vi "GetSensorValues.vi"(1 "Ref_BuiltInAccelerometer":T8={"DevStatus"={"status"=FALSE, "code"=0, "source"=""}, "Scaling"={"Gain (VoltsPerG)"=0.0, "Center Voltage"=0.0}, "Analog Channels"={"X-Axis"=enum."Invalid", "Y-Axis"=enum."Invalid", "Z-Axis"=enum."Invalid"}, "I2C Bus"=enum."Invalid", "SPI Bus"=enum."Invalid", "Accel Range"=0, "ADXL Axes"={"X-Axis"=FALSE, "Y-Axis"=FALSE, "Z-Axis"=FALSE}, "Handle"=0, "Device Address"=0, "Accel Type"=enum."Analog"} {"Device Address" format="%.0x"; "Accel Range" items=["+/- 2 g", "+/- 4 g", "+/- 8 g", "+/- 16 g"]}, 3 "Rear Prox Sensor":T6, 4 "Right Prox Sensor":T6, 5 "Left Prox Sensor":T6, 6 "Upper Pressure Transducer":T6, 8 "Ref_Compressor":T15, 9 "Front-Right Prox Sensor":T6, 10 "Ref_ElevatorEncoder":T1={"DeviceStatus"={"status"=FALSE, "code"=0, "source"=""}, "Type"=enum."PWM", "PWM"={"PWM Channel"=enum."Invalid", "DeadBand"={"Name"="", "maxPositivePwm"=0, "minPositivePwm"=0, "centerPwm"=0, "maxNegativePwm"=0, "minNegativePwm"=0, "angularRange"=0}}, "CAN"={"Device Number"=0, "SetOutput VI Ref"=variant, "GetOutput VI Ref"=variant, "Enable VI Ref"=variant, "Disable VI Ref"=variant, "Data"=variant}, "Invert"=FALSE, "DIO PWM"={"PWM \"Enable\" Channel"=enum."Invalid", "DIOChannel"=enum."Invalid", "PWM Rate"=0.0}}, 11 "Front-Left Prox Sensor":T6, 12 "Ref_ElevatorLimitSwitches":T1={"DeviceStatus"={"status"=FALSE, "code"=0, "source"=""}, "Type"=enum."PWM", "PWM"={"PWM Channel"=enum."Invalid", "DeadBand"={"Name"="", "maxPositivePwm"=0, "minPositivePwm"=0, "centerPwm"=0, "maxNegativePwm"=0, "minNegativePwm"=0, "angularRange"=0}}, "CAN"={"Device Number"=0, "SetOutput VI Ref"=variant, "GetOutput VI Ref"=variant, "Enable VI Ref"=variant, "Disable VI Ref"=variant, "Data"=variant}, "Invert"=FALSE, "DIO PWM"={"PWM \"Enable\" Channel"=enum."Invalid", "DIOChannel"=enum."Invalid", "PWM Rate"=0.0}}, 15 "Tank Pressure Transducer":T6, 19 "Ground Prox Sensor":T6, 20 "Ref_Drive 1R":T1, 21 "Ref_Drive 2R":T1, 22 "Ref_Drive 3L":T1, 23 "Ref_Drive 4L":T1, 24 "Ref_Drive 5L":T1, 26 "Ref_Drive 6R":T1) -> ()   [LabVIEW 2018]
uses:
  <vilib>/Rock Robotics/WPI/AnalogChannel/WPI_AnalogChannelDevRef.ctl
  <vilib>/Rock Robotics/SystemInterfaces/AI/FPGA_AIChannel.ctl
  <vilib>/Rock Robotics/WPI/Compressor/WPI_CompressorDevRef.ctl
  <vilib>/Rock Robotics/WPI/MotorControl/WPI_MotorControlDeviceRef.ctl
  <vilib>/Rock Robotics/WPI/MotorControl/WPI_MotorControlType.ctl
  <vilib>/Rock Robotics/SystemInterfaces/DIO/FPGA_DIOPWMChannel.ctl
  <vilib>/Rock Robotics/WPI/PWM/WPI_PWMDeadband.ctl
  <vilib>/Rock Robotics/SystemInterfaces/DIO/FPGA_DIOChannel.ctl
  <vilib>/Rock Robotics/WPI/Accelerometer/WPI_AccelerometerDevRef.ctl
  <vilib>/Rock Robotics/WPI/Accelerometer/WPI_AccelerometerScaling.ctl
  <vilib>/Rock Robotics/WPI/Accelerometer/WPI_AccelerometerAnalogChannels.ctl
  <vilib>/Rock Robotics/SystemInterfaces/i2clib/i2c_bus.ctl
  <vilib>/Rock Robotics/SystemInterfaces/spilib/spi_bus.ctl
  <vilib>/Rock Robotics/WPI/Accelerometer/ADXL345 Range.ctl
  <vilib>/Rock Robotics/WPI/Accelerometer/WPI_AccelerometerADXL345 Axes.ctl
  SensorReadings.vi
  RefNums_Actuators.vi
  RobotStates.vi
  Inputs_DriverStation.vi
  <vilib>/Rock Robotics/WPI/ThirdParty/Phoenix-LabVIEW/Motor Controller/Get/CTRE_Phoenix_MotorController_GetLimitSwitchStates.vi
  <vilib>/Rock Robotics/WPI/ThirdParty/Phoenix-LabVIEW/Motor Controller/Get/CTRE_Phoenix_MotorController_GetSelectedSensorData.vi
  <vilib>/gmath/NI_Gmath.lvlib
  <vilib>/Analysis/NI_AALBase.lvlib
panel:
  in  "Normal Elevator Std (A)":dbl=35.0
  in  "Off Ground Time (ms)":u32=100
  in  "On Ground Time (ms)":u32=1000
  in  "Ground Distance (in)":dbl=6.0
  in  "Plot Drive Encoder Data":bool
  in  "Tank Pressure Voltage Table":dbl[](array[numeric])=[0.4, 0.7, 0.9, 1.2, 1.4, 1.7, 1.9, 2.3, 2.5, 2.8, 3.0, 3.3] format="%_6g"
  in  "Tank Pressure PSI Table":dbl[](array[numeric])=[0.0, 10.0, 20.0, 30.0, 40.0, 50.0, 60.0, 70.0, 80.0, 90.0, 100.0, 115.0] format="%_6g"
  in  "LR Voltage Table":dbl[](array[numeric])=[0.43, 0.45, 0.47, 0.55, 0.6, 0.68, 0.72, 0.81, 0.86, 0.98, 1.13, 1.36, 1.53, 1.77, 1.99, 2.26, 2.52, 2.76] format="%_6g"
  in  "LR Distance Table":dbl[](array[numeric])=[150.661, 140.6, 133.7, 120.9, 110.1, 95.3, 90.1, 80.0, 73.7, 64.6, 55.9, 45.6, 40.2, 35.0, 29.6, 24.3, 19.6, 14.8] format="%_6g"
  in  "Suction Threshold (V)":dbl=0.1
  in  "SR Voltage Table":dbl[](array[numeric])=[3.15, 2.82, 2.51, 2.16, 1.92, 1.7, 1.49, 1.3, 1.12, 0.97, 0.87, 0.79, 0.72, 0.64, 0.61, 0.58, 0.52, 0.47, 0.46, 0.45, 0.43, 0.41] format="%_6g"
  in  "SR Distance Table":dbl[](array[numeric])=[4.6, 6.6, 8.3, 10.4, 12.2, 14.1, 16.5, 19.9, 23.6, 28.2, 32.6, 36.8, 40.9, 46.3, 49.9, 53.7, 58.3, 63.5, 67.5, 71.5, 75.1, 78.9] format="%_6g"
  out "Drive Encoder Velocities":cluster{dbl, dbl}(graph)
  # "*** Alpha was set to 6 inches ***"
  # "*** Beta was set to 12 inches ***"
  # "ADXL"
  # "Analog"
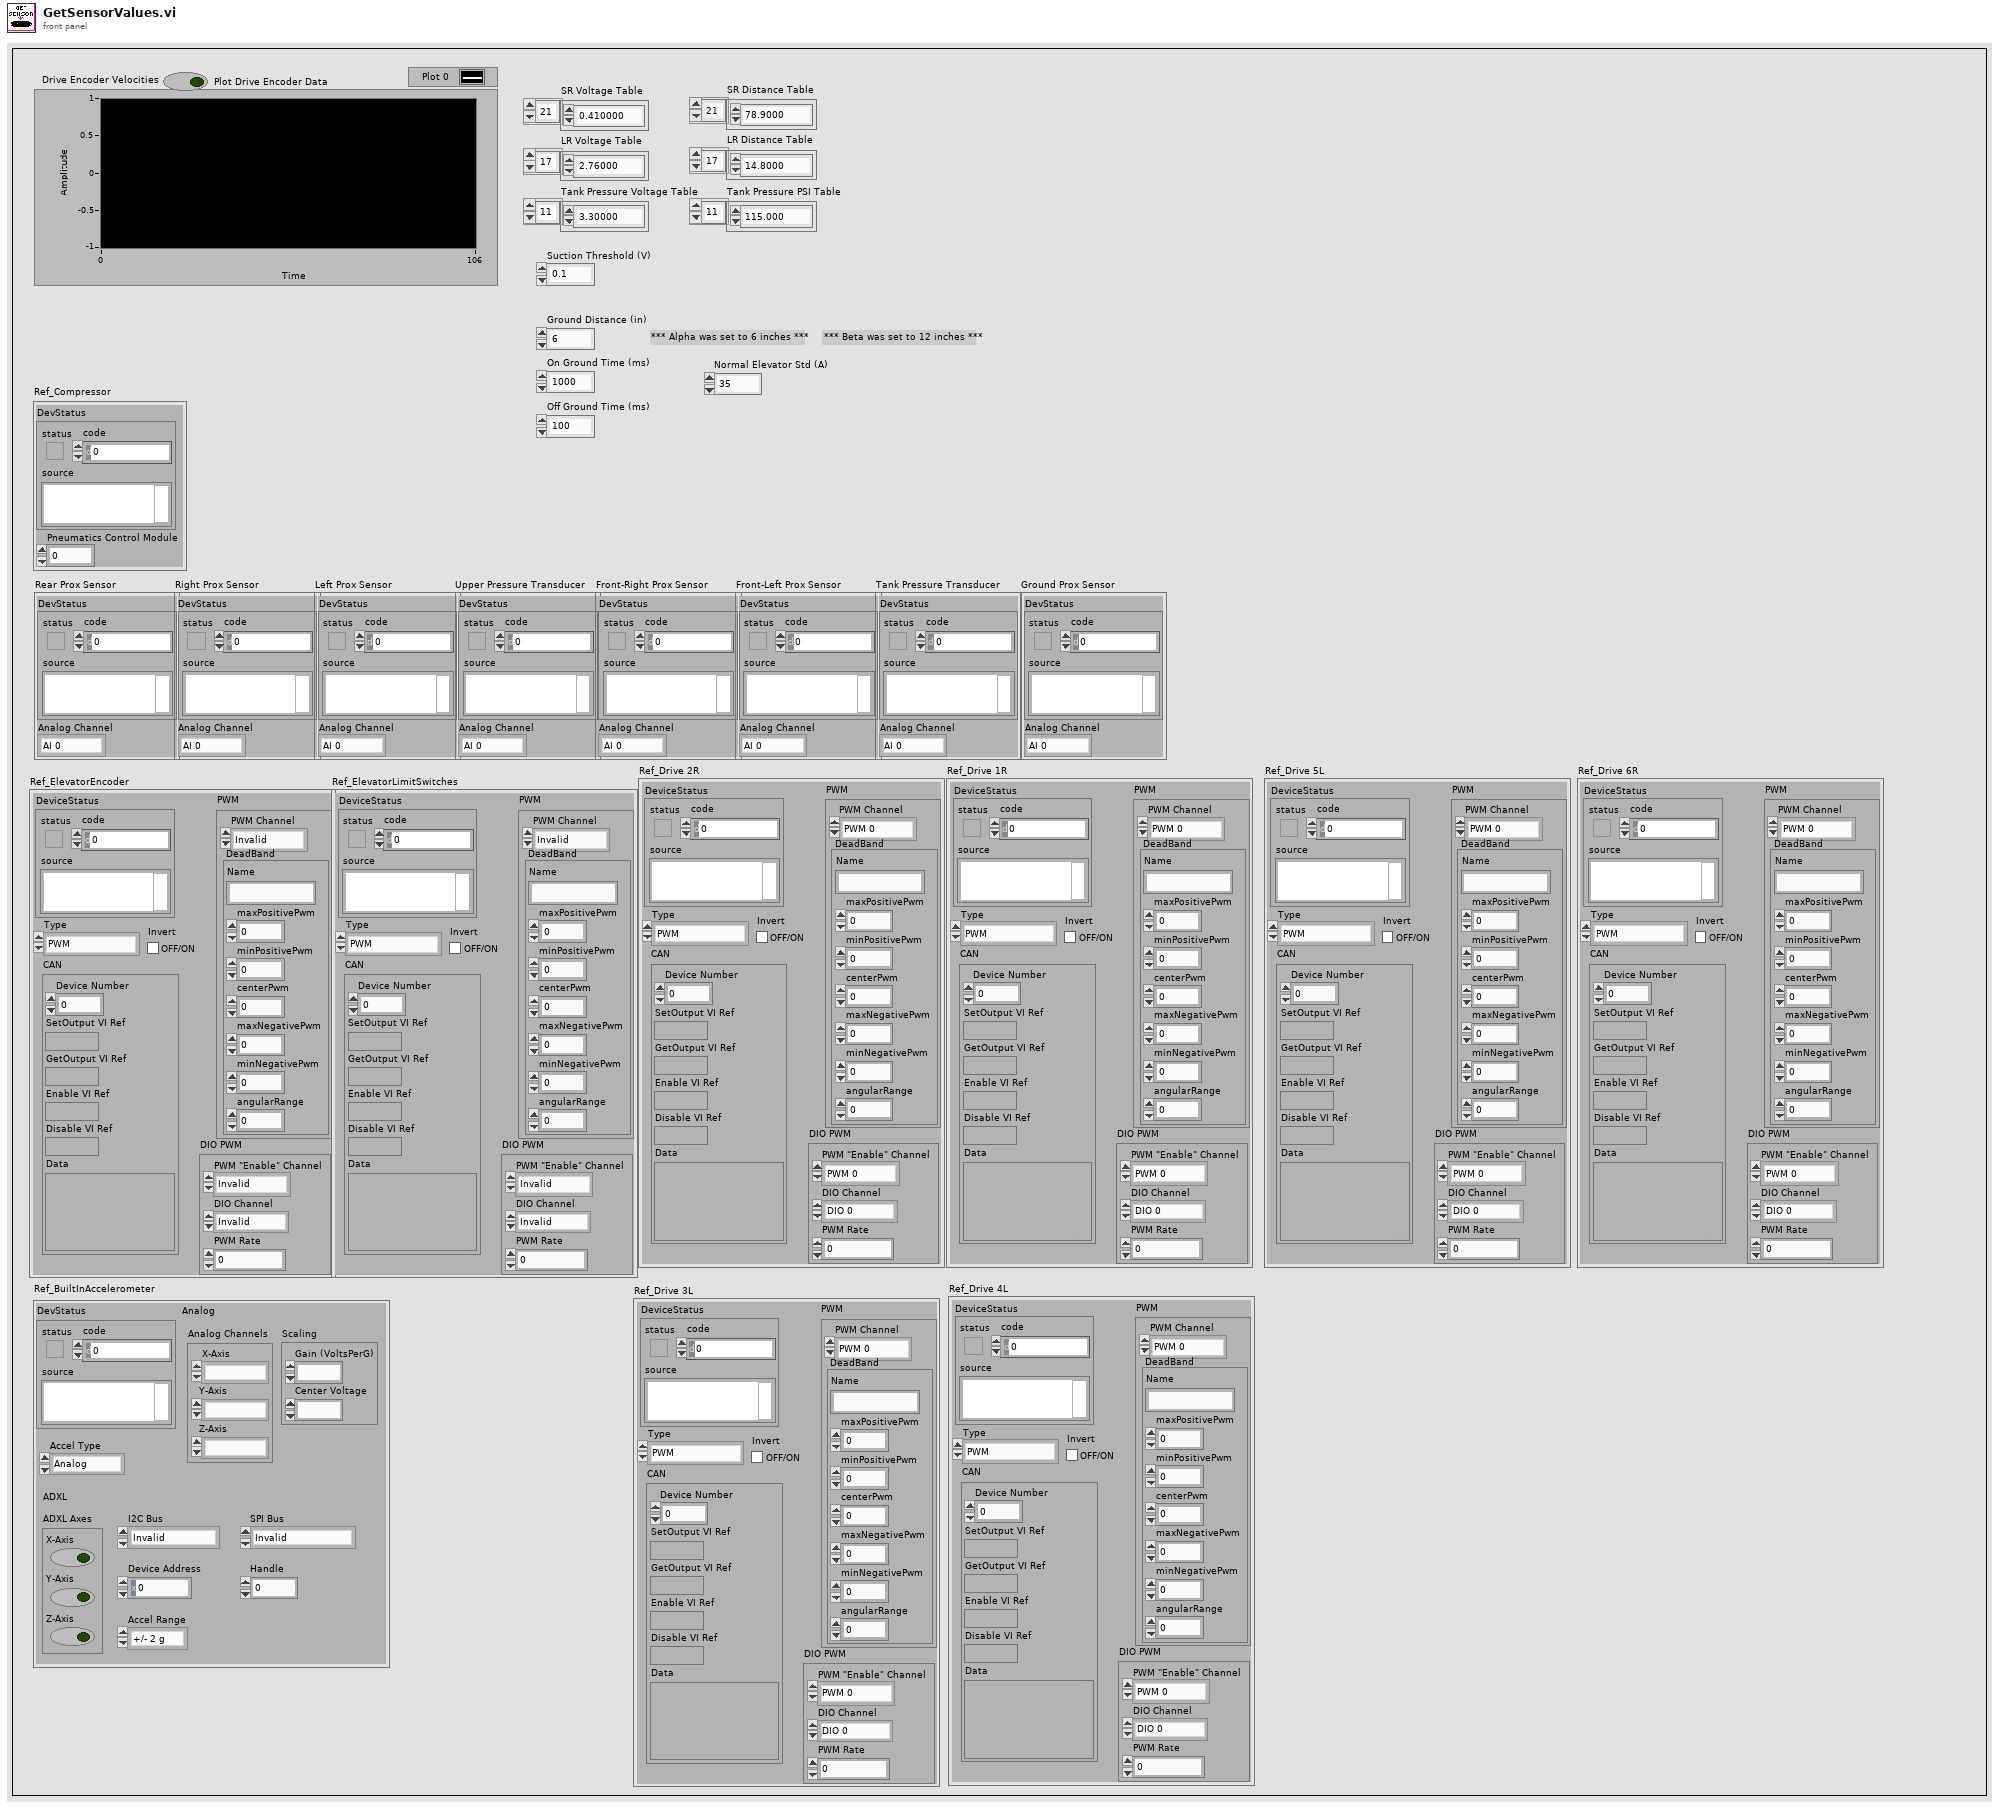
[diagram p1: front panel]
types:
  T1 = typedef "WPI_MotorControlDeviceRef.ctl" = cluster{"DeviceStatus":errorcluster, "Type":T2, "PWM":cluster{"PWM Channel":T3, "DeadBand":T4}, "CAN":cluster{"Device Number":u8, "SetOutput VI Ref":variant, "GetOutput VI Ref":variant, "Enable VI Ref":variant, "Disable VI Ref":variant, "Data":variant}, "Invert":bool, "DIO PWM":cluster{"PWM \"Enable\" Channel":T3, "DIOChannel":T5, "PWM Rate":dbl}}
  T2 = typedef "WPI_MotorControlType.ctl" = enum16{"PWM", "CAN", "DIO PWM"}
  T3 = typedef "FPGA_DIOPWMChannel.ctl" = enum8{"PWM 0", "PWM 1", "PWM 2", "PWM 3", "PWM 4", "PWM 5", "PWM 6", "PWM 7", "PWM 8", "PWM 9", "PWM MXP 0", "PWM MXP 1", "PWM MXP 2", "PWM MXP 3", "PWM MXP 4", "PWM MXP 5", "PWM MXP 6", "PWM MXP 7", "PWM MXP 8", "PWM MXP 9", "Invalid"}
  T4 = typedef "WPI_PWMDeadband.ctl" = cluster{"Name":string, "maxPositivePwm":i32, "minPositivePwm":i32, "centerPwm":i32, "maxNegativePwm":i32, "minNegativePwm":i32, "angularRange":u16}
  T5 = typedef "FPGA_DIOChannel.ctl" = enum8{"DIO 0", "DIO 1", "DIO 2", "DIO 3", "DIO 4", "DIO 5", "DIO 6", "DIO 7", "DIO 8", "DIO 9", "DIO MXP 0", "DIO MXP 1", "DIO MXP 2", "DIO MXP 3", "DIO MXP 4", "DIO MXP 5", "DIO MXP 6", "DIO MXP 7", "DIO MXP 8", "DIO MXP 9", "DIO MXP 10", "DIO MXP 11", "DIO MXP 12", "DIO MXP 13", "DIO MXP 14", "DIO MXP 15", "SPI Port CS1", "SPI Port CS2", "SPI Port CS3", "SPI Port MISO", "SPI Port MOSI", "Invalid"}
  T6 = typedef "WPI_AnalogChannelDevRef.ctl" = cluster{"DevStatus":errorcluster, "Analog Channel":T7}
  T7 = typedef "FPGA_AIChannel.ctl" = enum8{"AI 0", "AI 1", "AI 2", "AI 3", "AI MXP 0", "AI MXP 1", "AI MXP 2", "AI MXP 3", "Invalid"}
  T8 = typedef "WPI_AccelerometerDevRef.ctl" = cluster{"DevStatus":errorcluster, "Scaling":T9, "Analog Channels":T10, "I2C Bus":T11, "SPI Bus":T12, "Accel Range":T13, "ADXL Axes":T14, "Handle":i32, "Device Address":u8, "Accel Type":enum16{"Analog", "ADXL345 I2C", "ADXL345 SPI", "Internal", "ADXL362 SPI"}}
  T9 = typedef "WPI_AccelerometerScaling.ctl" = cluster{"Gain (VoltsPerG)":dbl, "Center Voltage":dbl}
  T10 = typedef "WPI_AccelerometerAnalogChannels.ctl" = cluster{"X-Axis":T7, "Y-Axis":T7, "Z-Axis":T7}
  T11 = typedef "i2c_bus.ctl" = enum16{"I2C On-Board", "I2C MXP", "Invalid"}
  T12 = typedef "spi_bus.ctl" = enum16{"SPI On-Board, CS0", "SPI On-Board, CS1", "SPI On-Board, CS2", "SPI On-Board, CS3", "SPI MXP", "Invalid"}
  T13 = typedef "ADXL345 Range.ctl" = u8
  T14 = typedef "WPI_AccelerometerADXL345 Axes.ctl" = cluster{"X-Axis":bool, "Y-Axis":bool, "Z-Axis":bool}
  T15 = typedef "WPI_CompressorDevRef.ctl" = cluster{"DevStatus":errorcluster, "Pneumatics Control Module":u8}
  T16 = cluster{"X-Axis":dbl, "Y-Axis":dbl, "Z-Axis":dbl}
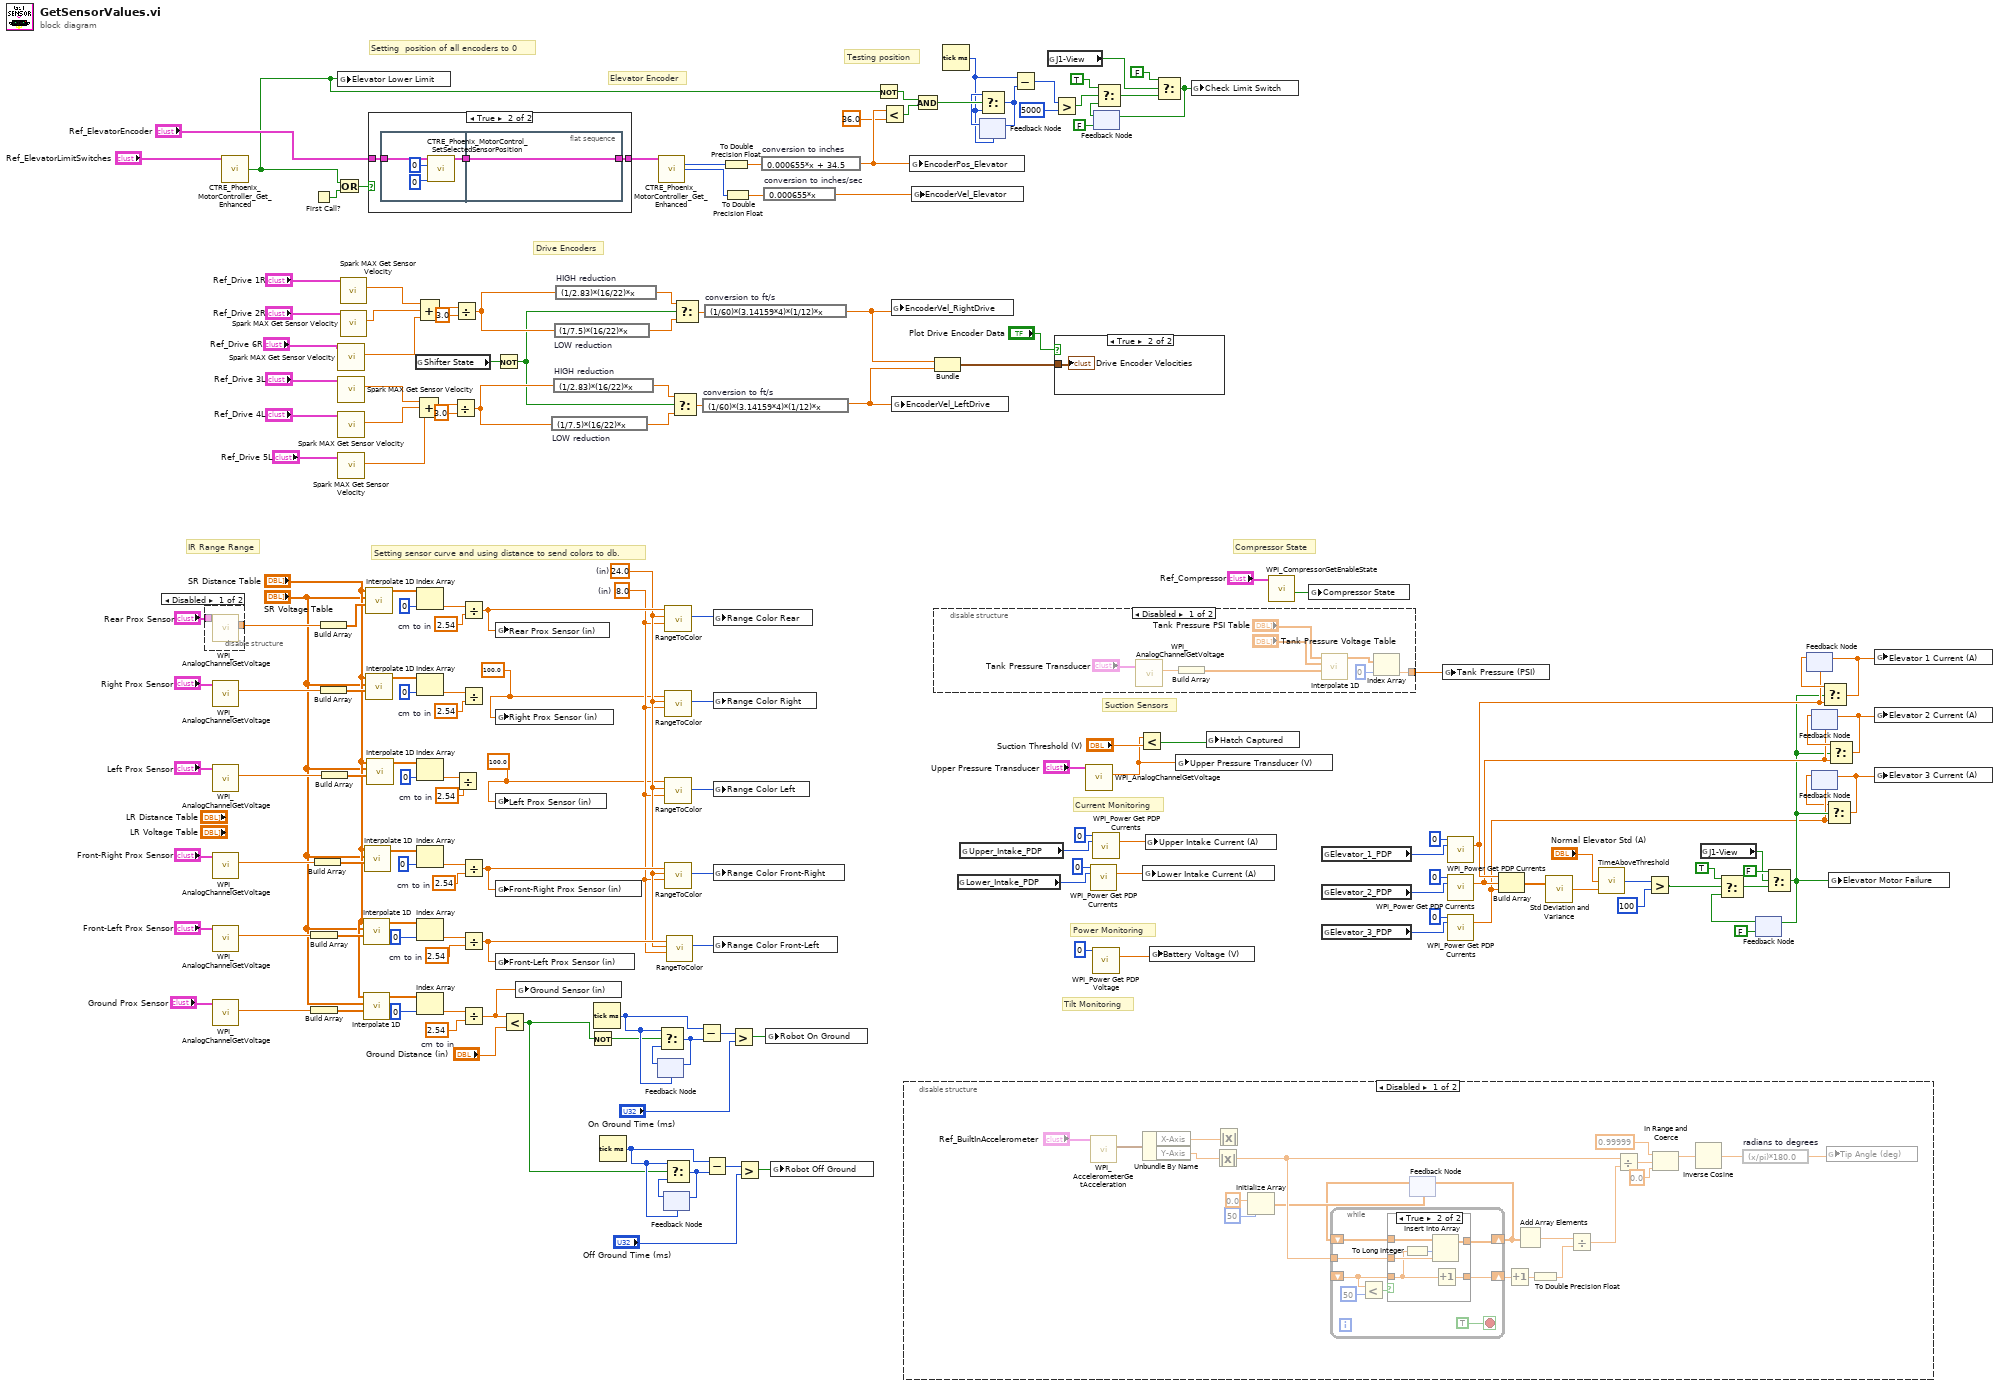
[diagram p0: block diagram]
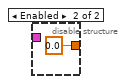
[diagram p2: hidden frame]
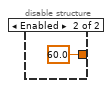
[diagram p6: hidden frame]
diagram:
  w5 = 100.0
  w6 = 100.0
  w76 = 2.54  # cm to in
  w133 = 2.54  # cm to in
  w126 = 8.0  # (in)
  w127 = 24.0  # (in)
  w150 = 2.54  # cm to in
  w156 = 2.54  # cm to in
  w163 = 2.54  # cm to in
  w170 = 2.54  # cm to in
  # "Elevator Encoder"
  # "Tilt Monitoring"
  # "Drive Encoders"
  # "Power Monitoring"
  # "Testing position"
  # "Setting  position of all encoders to 0"
  # "Setting sensor curve and using distance to send colors to db."
  # "Current Monitoring"
  # "Suction Sensors"
  # "Compressor State"
  # "IR Range Range"
  n1 = disable-structure shown="Disabled" {
    disable-tunnel: [w176 0.0 ("Voltage")] -> w174
    disable-tunnel: "Rear Prox Sensor" -> [w175 _]
    frame Disabled {
      n2 = call <vilib>:"WPI_AnalogChannelGetVoltage.vi"("AIDeviceRef"=w175) -> ("Voltage"=w176:dbl)  [unwired: 8 in, 2 out]
    }
    frame Enabled {
    }
  }
  n3 = call <vilib>:"WPI_AnalogChannelGetVoltage.vi"("AIDeviceRef"="Right Prox Sensor") -> ("Voltage"=w168:dbl)  [unwired: 8 in, 2 out]
  n4 = call <vilib>:"WPI_AnalogChannelGetVoltage.vi"("AIDeviceRef"="Left Prox Sensor") -> ("Voltage"=w161:dbl)  [unwired: 8 in, 2 out]
  n5 = call <vilib>:"WPI_AnalogChannelGetVoltage.vi"("AIDeviceRef"="Front-Right Prox Sensor") -> ("Voltage"=w138:dbl)  [unwired: 8 in, 2 out]
  n6 = call <vilib>:"WPI_AnalogChannelGetVoltage.vi"("AIDeviceRef"="Front-Left Prox Sensor") -> ("Voltage"=w131:dbl)  [unwired: 8 in, 2 out]
  n7 = call <vilib>:"WPI_AnalogChannelGetVoltage.vi"("AIDeviceRef"="Ground Prox Sensor") -> ("Voltage"=w75:dbl)  [unwired: 8 in, 2 out]
  n8 = call-poly <vilib>:"CTRE_Phoenix_MotorController_Get_Enhanced.vi"("PhoenixMotorControlDevRef"="Ref_ElevatorLimitSwitches") -> ("Reverse Limit Closed?"=w22:bool)  [unwired: 11 in, 3 out]
  n9 = First Call?() -> (First Call?: T/F=w80:bool)
  n10 = Build Array(w131) -> (w136:dbl[])
  n11 = Build Array(w75) -> (w79:dbl[])
  n12 = Build Array(w138) -> (w154:dbl[])
  n13 = Build Array(w174) -> (w148:dbl[])
  n14 = Build Array(w168) -> (w167:dbl[])
  n15 = Build Array(w161) -> (w160:dbl[])
  n16 = Or(x=w22, y=w80) -> (x .or. y?=w81:bool)
  n17 = global write "SensorReadings.vi" "Elevator Lower Limit"(w22) -> ()
  n18 = call <vilib>:"Spark MAX Get Sensor Velocity.vi"("MotorControlDevRef in"="Ref_Drive 6R") -> ("Sensor Velocity"=w2:dbl)  [unwired: 7 in, 3 out]
  n19 = call <vilib>:"Spark MAX Get Sensor Velocity.vi"("MotorControlDevRef in"="Ref_Drive 3L") -> ("Sensor Velocity"=w108:dbl)  [unwired: 7 in, 3 out]
  n20 = call <vilib>:"Spark MAX Get Sensor Velocity.vi"("MotorControlDevRef in"="Ref_Drive 4L") -> ("Sensor Velocity"=w107:dbl)  [unwired: 7 in, 3 out]
  n21 = call <vilib>:"Spark MAX Get Sensor Velocity.vi"("MotorControlDevRef in"="Ref_Drive 5L") -> ("Sensor Velocity"=w1:dbl)  [unwired: 7 in, 3 out]
  n22 = call <vilib>:"Spark MAX Get Sensor Velocity.vi"("MotorControlDevRef in"="Ref_Drive 1R") -> ("Sensor Velocity"=w113:dbl)  [unwired: 7 in, 3 out]
  n23 = call <vilib>:"Spark MAX Get Sensor Velocity.vi"("MotorControlDevRef in"="Ref_Drive 2R") -> ("Sensor Velocity"=w54:dbl)  [unwired: 7 in, 3 out]
  n24 = call <vilib>:"Interpolate 1D.vi"("xi"=w136, "X"="SR Voltage Table", "Y"="SR Distance Table") -> ("yi"=w130:dbl[])  [unwired: 6 in, 2 out]
  n25 = call <vilib>:"Interpolate 1D.vi"("xi"=w79, "X"="SR Voltage Table", "Y"="SR Distance Table") -> ("yi"=w74:dbl[])  [unwired: 6 in, 2 out]
  n26 = call <vilib>:"Interpolate 1D.vi"("xi"=w154, "X"="SR Voltage Table", "Y"="SR Distance Table") -> ("yi"=w151:dbl[])  [unwired: 6 in, 2 out]
  n27 = call <vilib>:"Interpolate 1D.vi"("xi"=w148, "X"="SR Voltage Table", "Y"="SR Distance Table") -> ("yi"=w171:dbl[])  [unwired: 6 in, 2 out]
  n28 = call <vilib>:"Interpolate 1D.vi"("xi"=w167, "X"="SR Voltage Table", "Y"="SR Distance Table") -> ("yi"=w164:dbl[])  [unwired: 6 in, 2 out]
  n29 = call <vilib>:"Interpolate 1D.vi"("xi"=w160, "X"="SR Voltage Table", "Y"="SR Distance Table") -> ("yi"=w157:dbl[])  [unwired: 6 in, 2 out]
  n30 = case shown="True" w81 {
    tunnel: "Ref_ElevatorEncoder" -> [w178 w181]
    tunnel: [w178 w179] -> w86
    frame False {
    }
    frame True {
      n31 = flat-sequence {
        tunnel: w181 -> [w185]
        tunnel: [w184] -> w180
        tunnel: [w186] -> w179
        tunnel: w180 -> [w186]
        frame #0 {
          n32 = call <vilib>:"CTRE_Phoenix_MotorControl_SetSelectedSensorPosition.vi"("pidLoopIdx"=u32 0, "New Sensor Position"=0, "PhoenixMotorControlDevRef"=w185) -> ("PhoenixMotorControlDevRef"=w184:T1)  [unwired: 7 in, 1 out]
        }
        frame #1 {
        }
      }
    }
  }
  n33 = global read "RobotStates.vi" "Shifter State"() -> (w100:bool)
  n34 = Index Array(array=w171, index=0) -> (element=w172:dbl)
  n35 = Index Array(array=w164, index=0) -> (element=w165:dbl)
  n36 = Index Array(array=w157, index=0) -> (element=w158:dbl)
  n37 = Index Array(array=w151, index=0) -> (element=w152:dbl)
  n38 = Index Array(array=w130, index=0) -> (element=w134:dbl)
  n39 = Index Array(array=w74, index=0) -> (element=w77:dbl)
  n40 = Compound Arithmetic op=ADD(w108, w107, w1) -> (w110:dbl)
  n41 = Compound Arithmetic op=ADD(w113, w54, w2) -> (w112:dbl)
  n42 = Divide(x=w110, y=3.0) -> (x/y=w101:dbl)
  n43 = Divide(x=w112, y=3.0) -> (x/y=w104:dbl)
  n44 = Divide(x=w158, y=w156) -> ()  [unwired: 1 out]
  n45 = Divide(x=w172, y=w170) -> (x/y=w147:dbl)
  n46 = Divide(x=w165, y=w163) -> ()  [unwired: 1 out]
  n47 = Divide(x=w152, y=w150) -> (x/y=w146:dbl)
  n48 = Divide(x=w134, y=w133) -> (x/y=w132:dbl)
  n49 = Divide(x=w77, y=w76) -> (x/y=w57:dbl)
  n50 = Not(x=w100) -> (.not. x?=w88:bool)
  n51 = global write "SensorReadings.vi" "Rear Prox Sensor (in)"(w147) -> ()
  n52 = global write "SensorReadings.vi" "Right Prox Sensor (in)"(w6) -> ()
  n53 = global write "SensorReadings.vi" "Left Prox Sensor (in)"(w5) -> ()
  n54 = global write "SensorReadings.vi" "Front-Right Prox Sensor (in)"(w146) -> ()
  n55 = global write "SensorReadings.vi" "Front-Left Prox Sensor (in)"(w132) -> ()
  n56 = Less?(x=w57, y="Ground Distance (in)") -> (x < y?=w56:bool)
  n57 = global write "SensorReadings.vi" "Ground Sensor (in)"(w57) -> ()
  n58 = expression code="(1/7.5)*(16/22)*x" "LOW reduction"(w101) -> (w102:dbl)
  n59 = expression code="(1/2.83)*(16/22)*x" "HIGH reduction"(w101) -> (w103:dbl)
  n60 = expression code="(1/7.5)*(16/22)*x" "LOW reduction"(w104) -> (w105:dbl)
  n61 = expression code="(1/2.83)*(16/22)*x" "HIGH reduction"(w104) -> (w106:dbl)
  n62 = Not(x=w56) -> (.not. x?=w55:bool)
  n63 = Tick Count (ms)() -> (millisecond timer value=w67:u32)
  n64 = Tick Count (ms)() -> (millisecond timer value=w62:u32)
  n65 = feedback #1(w67) -> (w69:u32)
  n66 = call-poly <vilib>:"CTRE_Phoenix_MotorController_Get_Enhanced.vi"("PhoenixMotorControlDevRef"=w86) -> ("Position (Raw Sensor Units)"=w85:i32, "Velocity (Raw Sensor Units per 100 ms)"=w83:i32)  [unwired: 11 in, 2 out]
  n67 = Select(t=w67, s=w55, f=w69) -> (s? t:f=w68:u32)
  n68 = feedback-in #1(w68) -> ()
  n69 = feedback #2(w62) -> (w64:u32)
  n70 = call "RangeToColor.vi"("Really Close (in)"=w126, "Close (in)"=w127, "Range (in)"=w147) -> ("Range Color"=w145:u32)  [unwired: 8 in]
  n71 = call "RangeToColor.vi"("Really Close (in)"=w126, "Close (in)"=w127, "Range (in)"=w6) -> ("Range Color"=w144:u32)  [unwired: 8 in]
  n72 = call "RangeToColor.vi"("Really Close (in)"=w126, "Close (in)"=w127, "Range (in)"=w5) -> ("Range Color"=w143:u32)  [unwired: 8 in]
  n73 = call "RangeToColor.vi"("Really Close (in)"=w126, "Close (in)"=w127, "Range (in)"=w146) -> ("Range Color"=w142:u32)  [unwired: 8 in]
  n74 = Select(t=w62, s=w56, f=w64) -> (s? t:f=w63:u32)
  n75 = feedback-in #2(w63) -> ()
  n76 = call "RangeToColor.vi"("Really Close (in)"=w126, "Close (in)"=w127, "Range (in)"=w132) -> ("Range Color"=w128:u32)  [unwired: 8 in]
  n77 = Select(t=w103, s=w88, f=w102) -> (s? t:f=w90:dbl)
  n78 = Select(t=w106, s=w88, f=w105) -> (s? t:f=w92:dbl)
  n79 = Subtract(x=w67, y=w68) -> (x-y=w66:u32)
  n80 = expression code="(1/60)*(3.14159*4)*(1/12)*x" "conversion to ft/s"(w90) -> (w89:dbl)
  n81 = Subtract(x=w62, y=w63) -> (x-y=w61:u32)
  n82 = expression code="(1/60)*(3.14159*4)*(1/12)*x" "conversion to ft/s"(w92) -> (w91:dbl)
  n83 = global write "SensorReadings.vi" "Range Color Rear"(w145) -> ()
  n84 = global write "SensorReadings.vi" "Range Color Right"(w144) -> ()
  n85 = global write "SensorReadings.vi" "Range Color Left"(w143) -> ()
  n86 = global write "SensorReadings.vi" "Range Color Front-Right"(w142) -> ()
  n87 = global write "SensorReadings.vi" "Range Color Front-Left"(w128) -> ()
  n88 = To Double Precision Float(number=w85) -> (double precision float=w87:dbl)
  n89 = To Double Precision Float(number=w83) -> (double precision float=w84:dbl)
  n90 = Greater?(x=w66, y="On Ground Time (ms)") -> (0:w65:bool)
  n91 = Greater?(x=w61, y="Off Ground Time (ms)") -> (0:w60:bool)
  n92 = expression code="0.000655*x + 34.5" "conversion to inches"(w87) -> (w25:dbl)
  n93 = expression code="0.000655*x" "conversion to inches/sec"(w84) -> (w82:dbl)
  n94 = global write "SensorReadings.vi" "Robot On Ground"(w65) -> ()
  n95 = global write "SensorReadings.vi" "Robot Off Ground"(w60) -> ()
  n96 = Not(x=w22) -> (.not. x?=w24:bool)
  n97 = Less?(x=w25, y=36.0) -> (x < y?=w23:bool)
  n98 = global write "SensorReadings.vi" "EncoderVel_RightDrive"(w91) -> ()
  n99 = global write "SensorReadings.vi" "EncoderVel_LeftDrive"(w89) -> ()
  n100 = disable-structure shown="Disabled" {
    frame Disabled {
      n101 = call <vilib>:"WPI_AccelerometerGetAcceleration.vi"("AccelerometerDevRef"="Ref_BuiltInAccelerometer") -> ("Accelerations"=w207:T16)  [unwired: 8 in, 2 out]
      n102 = Unbundle By Name(w207) -> ("X-Axis"=w205:dbl, "Y-Axis"=w204:dbl)
      n103 = Absolute Value(x=w204) -> (abs(x)=w195:dbl)
      n104 = Absolute Value(x=w205) -> ()  [unwired: 1 out]
      n105 = Initialize Array(0.0 ("element"), 50 ("dimension size")) -> (w192:dbl[])
      n106 = feedback #3(w192) -> (w191:dbl[])
      n107 = while {
        shift-right: [w213] -> w193
        shift-left: w191 -> [w214]
        tunnel: w195 -> [w208]
        shift-right: [w212] -> w198
        shift-left: _ -> [w210]
        stop <- TRUE stop-if-true
        n108 = Less?(x=w210, y=50) -> (x < y?=w211:bool)
        n109 = case shown="True" w211 {
          tunnel: w214 -> [w217 w223]
          tunnel: [w217 w222] -> w213
          tunnel: w208 -> [_ w221]
          tunnel: w210 -> [w216 w220]
          tunnel: [w216 w219] -> w212
          frame False {
          }
          frame True {
            n110 = To Long Integer(number=w220) -> (32bit integer=w218:i32)
            n111 = Insert Into Array(array=w223, index=w218, new element=w221) -> (w222:dbl[])
            n112 = Increment(x=w220) -> (x+1=w219:dbl)
          }
        }
      }
      n113 = feedback-in #3(w193) -> ()
      n114 = Increment(x=w198) -> (x+1=w197:dbl)
      n115 = Add Array Elements(numeric array=w193) -> (sum=w199:dbl)
      n116 = To Double Precision Float(number=w197) -> (double precision float=w196:dbl)
      n117 = Divide(x=w199, y=w196) -> (x/y=w194:dbl)
      n118 = Divide(x=w195, y=w194) -> (x/y=w190:dbl)
      n119 = In Range and Coerce(upper limit=0.99999, x=w190, lower limit=0.0) -> (coerced(x)=w189:dbl)  [unwired: 1 out]
      n120 = Inverse Cosine(1:w189) -> (0:w202:dbl)
      n121 = expression code="(x/pi)*180.0" "radians to degrees"(w202) -> (w203:dbl)
      n122 = global write "SensorReadings.vi" "Tip Angle (deg)"(w203) -> ()
    }
    frame Enabled {
    }
  }
  n123 = global write "SensorReadings.vi" "EncoderPos_Elevator"(w25) -> ()
  n124 = global write "SensorReadings.vi" "EncoderVel_Elevator"(w82) -> ()
  n125 = Compound Arithmetic op=AND(w24, w23) -> (w15:bool)
  n126 = disable-structure shown="Disabled" {
    disable-tunnel: [w225 60.0 ("Tank Pressure (PSI)")] -> w118
    frame Disabled {
      n127 = call <vilib>:"WPI_AnalogChannelGetVoltage.vi"("AIDeviceRef"="Tank Pressure Transducer") -> ("Voltage"=w224:dbl)  [unwired: 8 in, 2 out]
      n128 = Build Array(w224) -> (w226:dbl[])
      n129 = call <vilib>:"Interpolate 1D.vi"("xi"=w226, "X"="Tank Pressure Voltage Table", "Y"="Tank Pressure PSI Table") -> ("yi"=w229:dbl[])  [unwired: 6 in, 2 out]
      n130 = Index Array(array=w229, index=0) -> (element=w225:dbl)
    }
    frame Enabled {
    }
  }
  n131 = Bundle(w91, w89) -> (w99:cluster{dbl, dbl})  [unwired: 1 in]
  n132 = Tick Count (ms)() -> (millisecond timer value=w9:u32)
  n133 = global read "RefNums_Actuators.vi" "Lower_Intake_PDP"() -> (w121:i32)
  n134 = global read "RefNums_Actuators.vi" "Upper_Intake_PDP"() -> (w124:i32)
  n135 = feedback #4(w9) -> (w14:u32)
  n136 = Select(t=w14, s=w15, f=w9) -> (s? t:f=w10:u32)
  n137 = feedback-in #4(w10) -> ()
  n138 = Subtract(x=w9, y=w10) -> (x-y=w8:u32)
  n139 = global read "Inputs_DriverStation.vi" "J1-View"() -> (w16:bool)
  n140 = Greater?(x=w8, y=u32 5000) -> (0:w11:bool)
  n141 = case shown="True" "Plot Drive Encoder Data" {
    tunnel: w99 -> [_ w233]
    frame False {
    }
    frame True {
      "Drive Encoder Velocities" <- w233
    }
  }
  n142 = call <vilib>:"WPI_AnalogChannelGetVoltage.vi"("AIDeviceRef"="Upper Pressure Transducer") -> ("Voltage"=w119:dbl)  [unwired: 8 in, 2 out]
  n143 = call <vilib>:"WPI_Power Get PDP Currents.vi"("Power Distribution Panel (0)"=u8 0, "PDP Channel"=w121) -> ("current (A)"=w120:dbl)  [unwired: 11 in, 2 out]
  n144 = call <vilib>:"WPI_Power Get PDP Currents.vi"("Power Distribution Panel (0)"=u8 0, "PDP Channel"=w124) -> ("current (A)"=w123:dbl)  [unwired: 11 in, 2 out]
  n145 = call <vilib>:"WPI_Power Get PDP Voltage.vi"("Power Distribution Panel (0)"=u8 0) -> ("voltage (V)"=w116:dbl)  [unwired: 13 in, 1 out]
  n146 = feedback #5(FALSE) -> (w21:bool)
  n147 = Select(t=TRUE, s=w11, f=w21) -> (s? t:f=w18:bool)
  n148 = Less?(x=w119, y="Suction Threshold (V)") -> (x < y?=w93:bool)
  n149 = global write "SensorReadings.vi" "Lower Intake Current (A)"(w120) -> ()
  n150 = global write "SensorReadings.vi" "Upper Intake Current (A)"(w123) -> ()
  n151 = global write "SensorReadings.vi" "Battery Voltage (V)"(w116) -> ()
  n152 = Select(t=FALSE, s=w16, f=w18) -> (s? t:f=w7:bool)
  n153 = feedback-in #5(w7) -> ()
  n154 = global write "SensorReadings.vi" "Upper Pressure Transducer (V)"(w119) -> ()
  n155 = global write "RobotStates.vi" "Check Limit Switch"(w7) -> ()
  n156 = global write "SensorReadings.vi" "Hatch Captured"(w93) -> ()
  n157 = call <vilib>:"WPI_CompressorGetEnableState.vi"("CompressorDevRef"="Ref_Compressor") -> ("Compressor Running"=w140:bool)  [unwired: 7 in, 3 out]
  n158 = global write "RobotStates.vi" "Compressor State"(w140) -> ()
  n159 = global read "RefNums_Actuators.vi" "Elevator_1_PDP"() -> (w52:i32)
  n160 = global read "RefNums_Actuators.vi" "Elevator_2_PDP"() -> (w50:i32)
  n161 = global read "RefNums_Actuators.vi" "Elevator_3_PDP"() -> (w48:i32)
  n162 = global write "SensorReadings.vi" "Tank Pressure (PSI)"(w118) -> ()
  n163 = call <vilib>:"WPI_Power Get PDP Currents.vi"("Power Distribution Panel (0)"=u8 0, "PDP Channel"=w52) -> ("current (A)"=w34:dbl)  [unwired: 11 in, 2 out]
  n164 = call <vilib>:"WPI_Power Get PDP Currents.vi"("Power Distribution Panel (0)"=u8 0, "PDP Channel"=w50) -> ("current (A)"=w31:dbl)  [unwired: 11 in, 2 out]
  n165 = call <vilib>:"WPI_Power Get PDP Currents.vi"("Power Distribution Panel (0)"=u8 0, "PDP Channel"=w48) -> ("current (A)"=w28:dbl)  [unwired: 11 in, 2 out]
  n166 = Build Array(w34, w31, w28) -> (w47:dbl[])
  n167 = call <vilib>:"Std Deviation and Variance.vi"("X"=w47) -> ("standard deviation"=w46:dbl)  [unwired: 1 in, 2 out]
  n168 = call "TimeAboveThreshold.vi"("Current Value"=w46, "Threshold"="Normal Elevator Std (A)") -> ("Time Above"=w44:u32)  [unwired: 3 in]
  n169 = Greater?(x=w44, y=u32 100) -> (0:w36:bool)
  n170 = global read "Inputs_DriverStation.vi" "J1-View"() -> (w37:bool)
  n171 = feedback #6(FALSE) -> (w41:bool)
  n172 = Select(t=TRUE, s=w36, f=w41) -> (s? t:f=w39:bool)
  n173 = Select(t=FALSE, s=w37, f=w39) -> (s? t:f=w29:bool)
  n174 = feedback-in #6(w29) -> ()
  n175 = feedback #7(w34) -> (w35:dbl)
  n176 = feedback #8(w31) -> (w32:dbl)
  n177 = feedback #9(w28) -> (w26:dbl)
  n178 = Select(t=w35, s=w29, f=w34) -> (s? t:f=w33:dbl)
  n179 = feedback-in #7(w33) -> ()
  n180 = Select(t=w26, s=w29, f=w28) -> (s? t:f=w27:dbl)
  n181 = feedback-in #9(w27) -> ()
  n182 = Select(t=w32, s=w29, f=w31) -> (s? t:f=w30:dbl)
  n183 = feedback-in #8(w30) -> ()
  n184 = global write "RobotStates.vi" "Elevator Motor Failure"(w29) -> ()
  n185 = global write "SensorReadings.vi" "Elevator 1 Current (A)"(w33) -> ()
  n186 = global write "SensorReadings.vi" "Elevator 2 Current (A)"(w30) -> ()
  n187 = global write "SensorReadings.vi" "Elevator 3 Current (A)"(w27) -> ()
